vi "LoadObserverControlMatrix_HystSatDrift.vi"(10 "ControlParams-ss-xy":T1={"umax"=3.0, "Ns_obs/cntrl"=0, "du_max"=0.0, "Nbar"=0.0, "Nhyst"=0, "Nsat"=0, "Ndrift+1"=0, "Ki-y"=0.01, "Ns_xff+1"=0, "Ns_yff+1"=0, "Ns_Dx+1"=0, "Ns_Dy+1"=0, "Ki-x"=0.01}) -> (2 "SS FIFO TimeOut?":bool, 3 "ControlParams-ss-xy 2":T1={"umax"=3.0, "Ns_obs/cntrl"=0, "du_max"=0.0, "Nbar"=0.0, "Nhyst"=0, "Nsat"=0, "Ndrift+1"=0, "Ki-y"=0.01, "Ns_xff+1"=0, "Ns_yff+1"=0, "Ns_Dx+1"=0, "Ns_Dy+1"=0, "Ki-x"=0.01})   [LabVIEW 2017]
uses:
  typeDefs/FXPControlParams-ss-xy.ctl
  <vilib>/Platform/TimedLoop/XDataNode/timing_clust.ctl
  <vilib>/Platform/TimedLoop/XDataNode/nitl_modes.ctl
  <vilib>/Platform/TimedLoop/XDataNode/wakeup.ctl
  typeDefs/Bz_bram.ctl
  typeDefs/Lz_bram.ctl
  typeDefs/Kz_bram.ctl
  typeDefs/A_as_vec_bram.ctl
  <vilib>/rvi/interface/RandomDataEmulation/niFpgaRandomDataHandleErrors.vi
  <vilib>/rvi/DataTransferAndStorage/Container/Common/niFpgaContainerExecOnDevCompGetState.vi
  <vilib>/rvi/Emulation/niFpgaEmulationIsFPGAContextNoSignature.vi
  <vilib>/rvi/DataTransferAndStorage/Container/Common/niFpgaContainerGetUniqueNameForEmu.vi
  <vilib>/rvi/Emulation/niFpgaProcessEmulError.vi
  <vilib>/rvi/Emulation/niFpgaSctlEmulationGetInTimedLoop.vi
  <vilib>/rvi/errors/nirviReportUnexpectedCaseInternalError (U32).vi
  <vilib>/rvi/Memory/Memory_Emulation/niFpgaMemoryEmulationCacheClearOnFirstRun.vi
  <vilib>/rvi/Memory/Memory_Emulation/nirvimemoryEmulationManagerCache_MakeExclusive.vi
  <vilib>/rvi/Memory/Memory_Emulation/niFpgaMemoryEmulationValidateCache.vi
  <vilib>/rvi/Memory/Memory_Emulation/nirvimemoryEmulationManagerCache_InsertValue.vi
  <vilib>/Utility/error.llb/Clear Errors.vi
  <vilib>/rvi/Memory/Memory_Emulation/nirvimemoryEmulationManagerCache_ReleaseExclusive.vi
  <vilib>/rvi/Memory/Memory_Emulation/nirvimemoryEmulationManagerCache_GetValue.vi
  <vilib>/rvi/Memory/Memory_Emulation/nirvimemoryEmulationManagerCache_SetValue.vi
  <vilib>/rvi/Emulation/niFpgaSctlEmulationResourceMgr.vi
  <vilib>/rvi/Emulation/niFpgaEmulationReportErrorSimple.vi
  <vilib>/rvi/Emulation/niFpgaGetClockAttributes.vi
  <vilib>/rvi/Emulation/niFpgaCriticalErrorInLSC.vi
  <vilib>/rvi/Memory/Memory_Emulation/nirvimemoryFastEmulation.vi
  <vilib>/rvi/Memory/Memory_Emulation/nirvimemoryEmulation.vi
  <vilib>/rvi/DataTransferAndStorage/Container/XNode/niFpgaContainer.xnode
  <vilib>/rvi/interface/RandomDataEmulation/nirviRandomDataFpgaReadWriteTemplate.vi
  <vilib>/rvi/Memory/Memory_Emulation/niFpgaMemoryEmulationRefIn.vi
  <vilib>/Platform/TimedLoop/XDataNode/XDataNode.xnode
  <vilib>/Platform/TimedLoop/XDataNode/XDNodeRunTimeDep.lvlib
panel:
  # "NOTE: Ns is the number of states in the plant. The number of states in the \nobserver is Ns+1. Thus, for B, L, C, and A, we use NS+1. For K and Xss, we use Ns\nbecause the controller does not operate on the disturbance state, Xd."
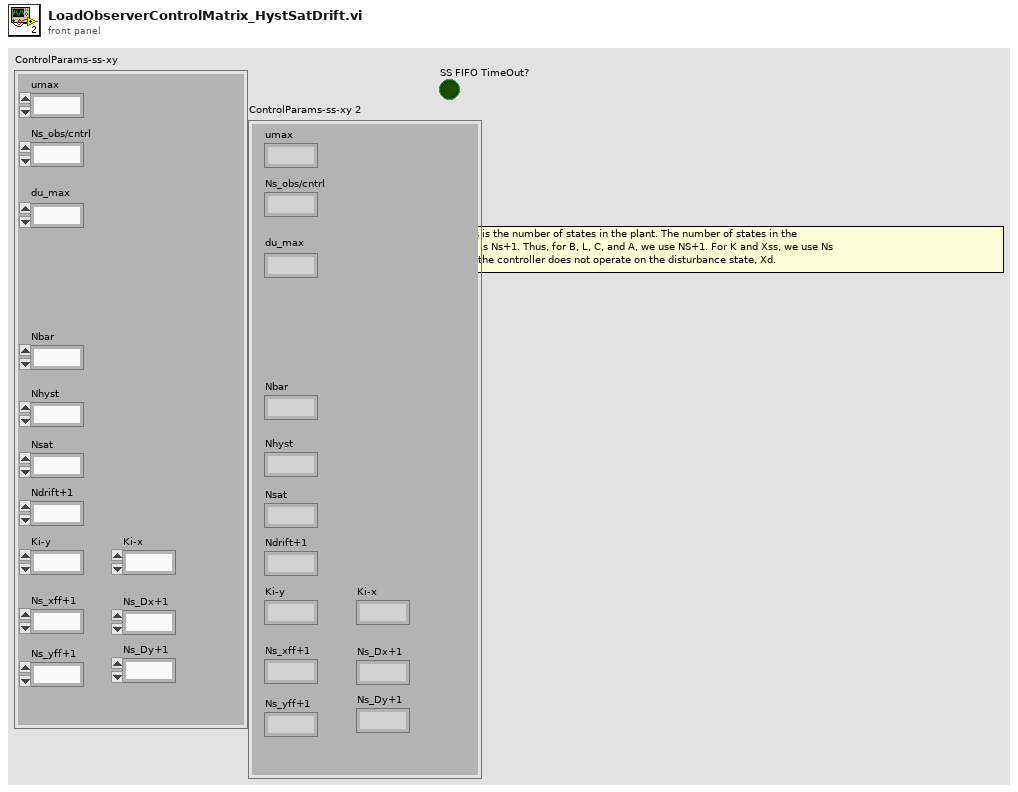
[diagram p1: front panel]
types:
  T1 = typedef "FXPControlParams-ss-xy.ctl" = cluster{"umax":fxp<+/-,18,5>, "Ns_obs/cntrl":u8, "du_max":fxp<+/-,18,5>, "Nbar":fxp<+/-,32,5>, "Nhyst":u8, "Nsat":u8, "Ndrift+1":u8, "Ki-y":sgl, "Ns_xff+1":u8, "Ns_yff+1":u8, "Ns_Dx+1":u8, "Ns_Dy+1":u8, "Ki-x":sgl}
  T2 = typedef "Bz_bram.ctl" = refnum<k21>
  T3 = typedef "Lz_bram.ctl" = refnum<k21>
  T4 = typedef "Kz_bram.ctl" = refnum<k21>
  T5 = typedef "A_as_vec_bram.ctl" = refnum<k21>
  T6 = typedef "XDNodeRunTimeDep.lvlib/timing_clust.ctl" = cluster{"Expected End [f-1]":u64, "Actual End [f-1]":u64, "Finished Late? [f-1]":bool, "Expected End [i-1]":u64, "Actual End [i-1]":u64, "Finished Late? [i-1]":bool, "Expected Start [i]":u64, "Actual Start [i]":u64, "Expected Start [f]":u64, "Actual Start [f]":u64, "Source Name":string, "Structure Name":string, "Period":i64, "Deadline":i64, "Offset":i64, "Start":i64, "Priority":i32, "Timeout":i32, "Mode":T7, "Wakeup Reason":T8, "Error":errorcluster, "Source Type":string, "Secondary Source Type":string, "Global End Time":u64, "Global Start Time":u64, "Frame Duration":u64, "Iteration Duration":u64, "Assigned CPU":i32, "I/O Scan Engine Mode":u32}
  T7 = typedef "XDNodeRunTimeDep.lvlib/nitl_modes.ctl" = enum32{"No Change", "Process missed periods, maintain original phase", "Discard missed periods, maintain original phase", "Process missed periods, ignore original phase", "Discard missed periods, ignore original phase"}
  T8 = typedef "XDNodeRunTimeDep.lvlib/wakeup.ctl" = enum32{"Normal", "Aborted", "Asynchronous wakeup", "Timing source error", "Timed loop error", "Timeout"}
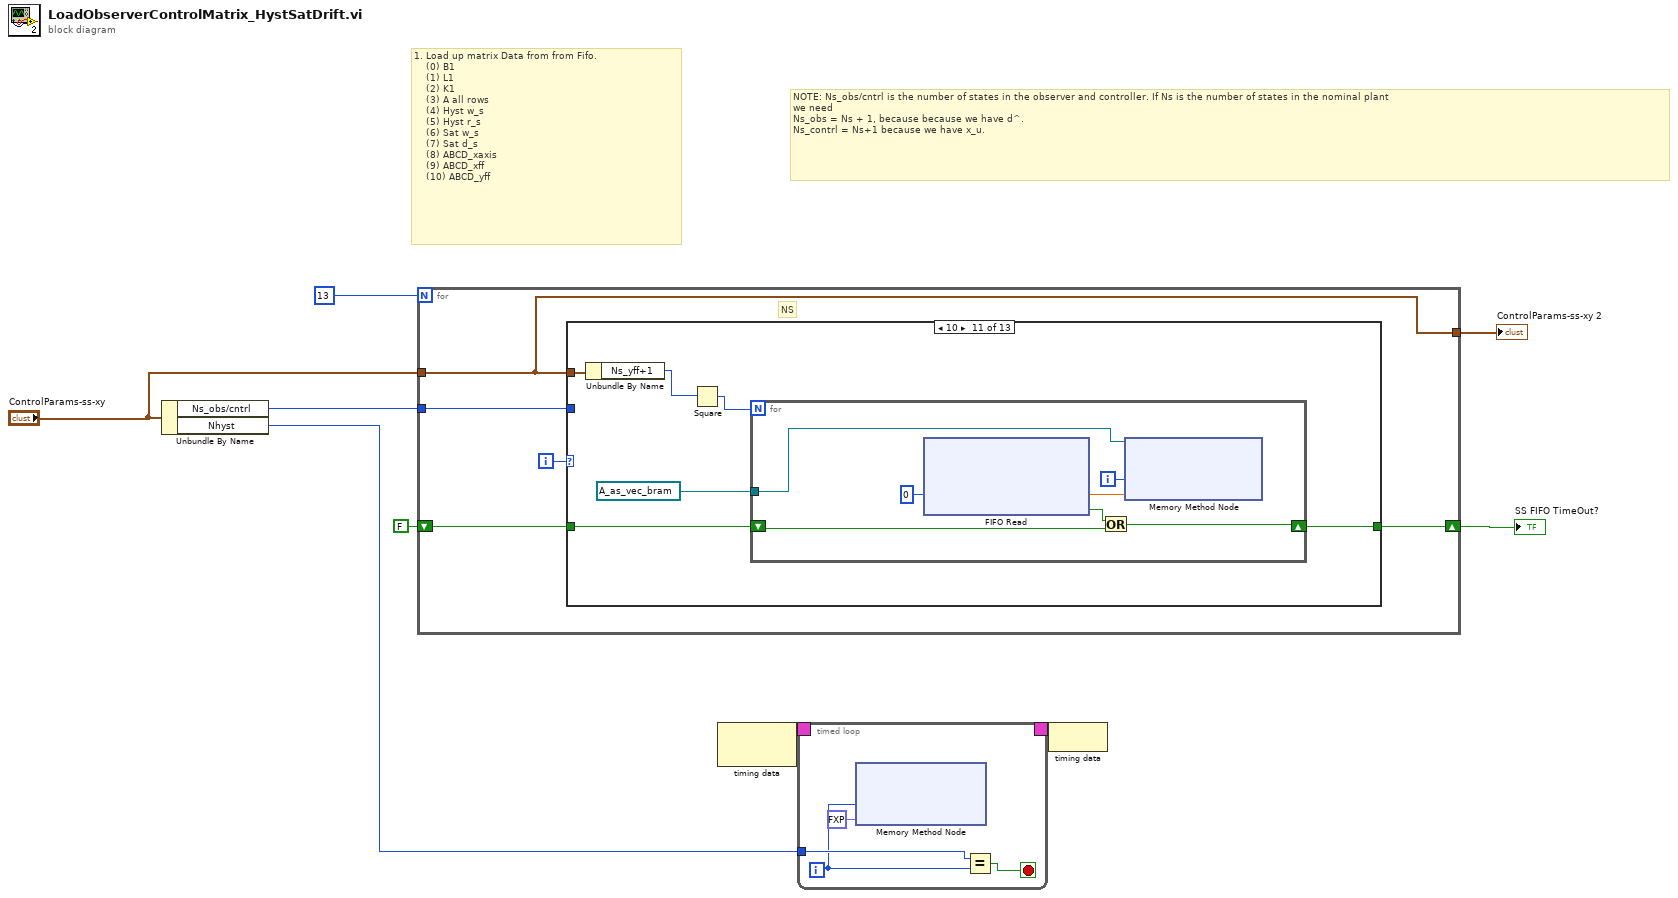
[diagram p0: block diagram]
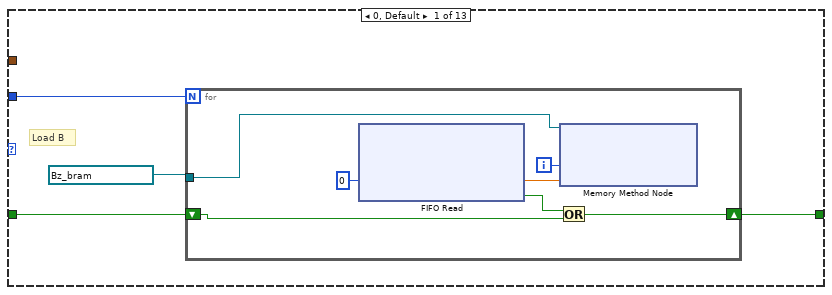
[diagram p2: hidden frame]
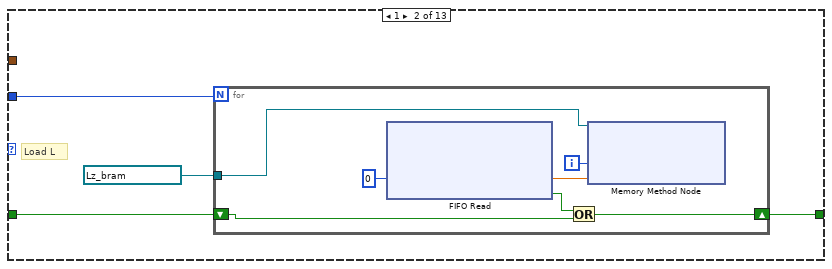
[diagram p3: hidden frame]
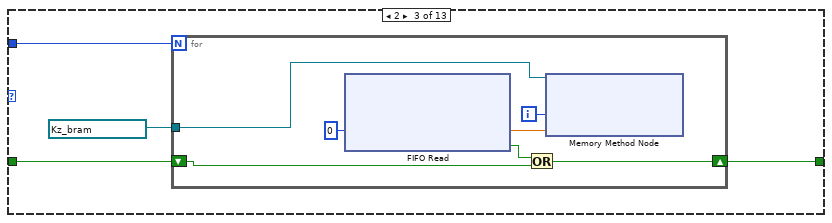
[diagram p4: hidden frame]
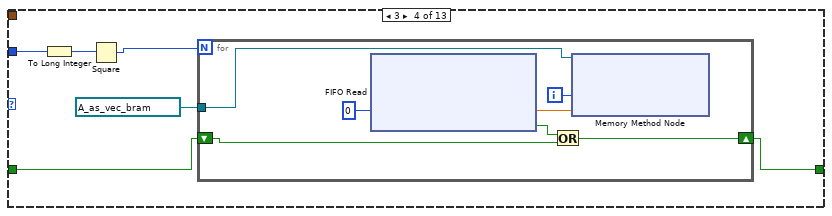
[diagram p5: hidden frame]
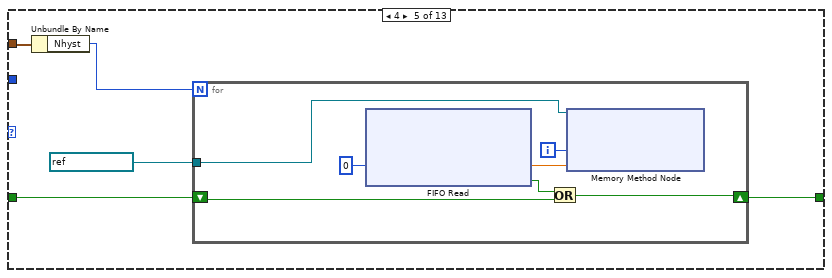
[diagram p6: hidden frame]
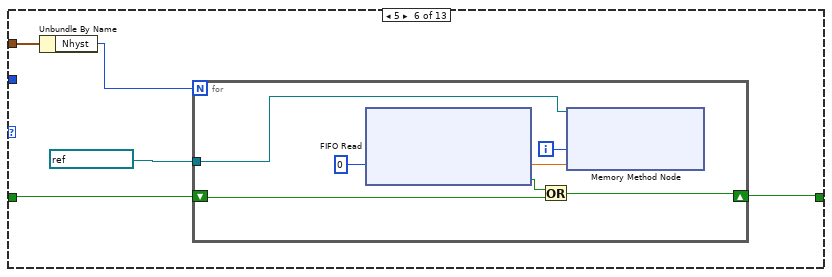
[diagram p7: hidden frame]
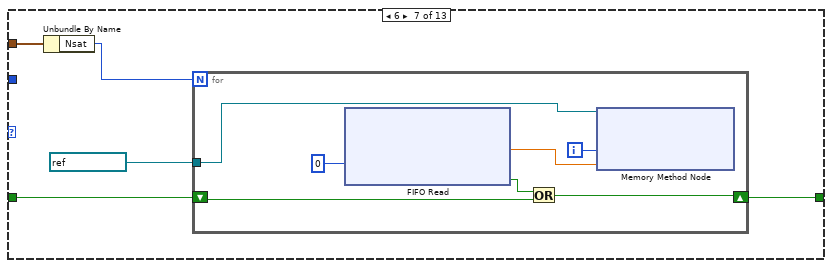
[diagram p8: hidden frame]
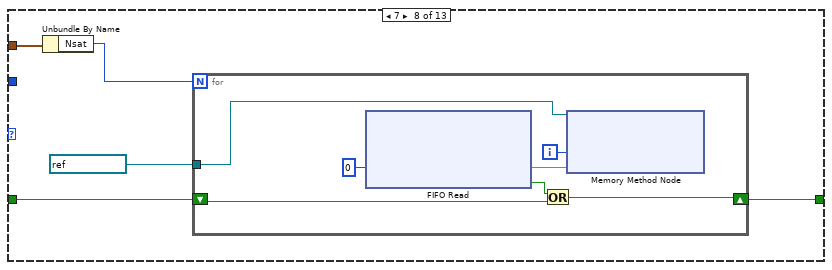
[diagram p9: hidden frame]
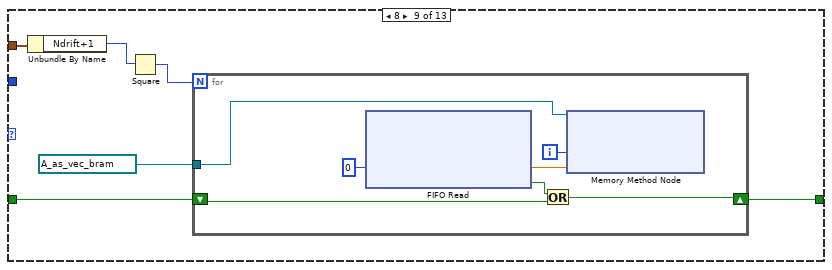
[diagram p10: hidden frame]
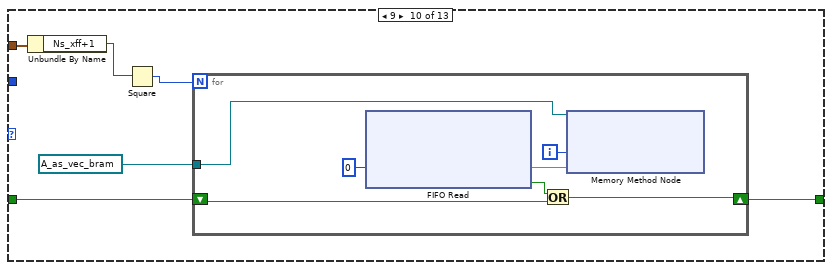
[diagram p11: hidden frame]
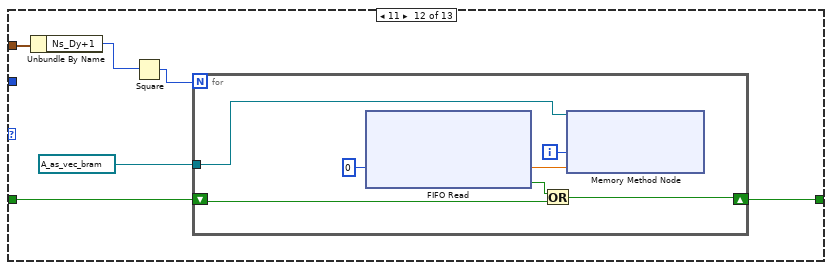
[diagram p12: hidden frame]
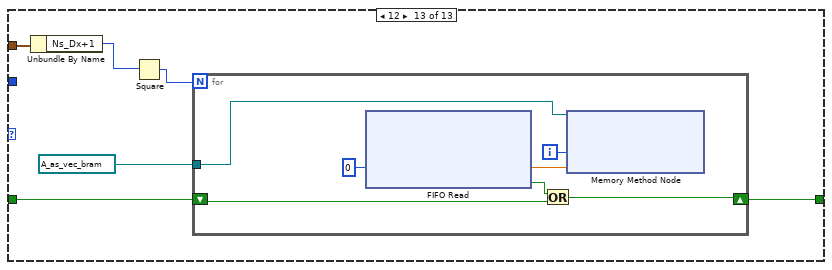
[diagram p13: hidden frame]
diagram:
  # "NOTE: Ns_obs/cntrl is the number of states in the observer and controller. If Ns is the number of states in the nominal plant\nwe need\nNs_obs = Ns + 1, because because we have d^. \nNs_contrl = Ns+1 because we have x_u."
  # "1. Load up matrix Data from from Fifo.\n    (0) B1\n    (1) L1\n    (2) K1 \n    (3) A all rows\n    (4) Hyst w_s\n    (5) Hyst r_s\n    (6) Sat w_s\n    (7) Sat d_s\n    (8) ABCD_xaxis\n    (9) ABCD_xff\n    (10) ABCD_yff"
  n1 = Unbundle By Name("ControlParams-ss-xy") -> ("Ns_obs/cntrl"=w4:u8, "Nhyst"=w3:u8)
  n2 = for {
    N: i16 13 -> [_]
    tunnel: w4 -> [w13]
    shift-right: [w11] -> w7
    shift-left: FALSE -> [w12]
    tunnel: "ControlParams-ss-xy" -> [w10]
    tunnel: [w10] -> w1
    i -> [w14]
    # "NS"
    n3 = case shown="10" w14 {
      tunnel: w13 -> [w18 w26 w40 w49 _ _ _ _ _ _ _ _ _]
      tunnel: w12 -> [w16 w28 w37 w50 w64 w76 w88 w100 w113 w126 w139 w152 w165]
      tunnel: [w15 w27 w38 w51 w65 w77 w89 w101 w114 w127 w140 w153 w166] -> w11
      tunnel: w10 -> [_ _ _ _ w62 w74 w86 w98 w111 w124 w137 w150 w163]
      frame 0, Default {
        # "Load B"
        n4 = for {
          N: w18 -> [_]
          tunnel: T2 "Bz_FXP_col1" ("Memory") -> [w23]
          shift-right: [w20] -> w15
          shift-left: w16 -> [w19]
          i -> [w22]
          n5 = xnode ("FIFO Read")("Timeout"=i16 0) -> ("Element"=w25:sgl, "Timed Out?"=w21:bool)  [unwired: 1 in, 1 out]
          n6 = Or(x=w21, y=w19) -> (x .or. y?=w20:bool)
          n7 = xnode ("Memory Method Node")("Address"=w22, "Data"=w25, "Memory In"=w23) -> ()  [unwired: 1 out]
        }
      }
      frame 1 {
        # "Load L"
        n8 = for {
          N: w26 -> [_]
          tunnel: T3 "L_FXP_col1" ("Memory") -> [w34]
          shift-right: [w31] -> w27
          shift-left: w28 -> [w30]
          i -> [w33]
          n9 = xnode ("FIFO Read")("Timeout"=i16 0) -> ("Element"=w36:sgl, "Timed Out?"=w32:bool)  [unwired: 1 in, 1 out]
          n10 = Or(x=w32, y=w30) -> (x .or. y?=w31:bool)
          n11 = xnode ("Memory Method Node")("Address"=w33, "Data"=w36, "Memory In"=w34) -> ()  [unwired: 1 out]
        }
      }
      frame 2 {
        n12 = for {
          N: w40 -> [_]
          tunnel: T4 "K_FXP_row1" ("Memory") -> [w45]
          shift-right: [w42] -> w38
          shift-left: w37 -> [w41]
          i -> [w44]
          n13 = xnode ("FIFO Read")("Timeout"=i16 0) -> ("Element"=w47:sgl, "Timed Out?"=w43:bool)  [unwired: 1 in, 1 out]
          n14 = Or(x=w43, y=w41) -> (x .or. y?=w42:bool)
          n15 = xnode ("Memory Method Node")("Address"=w44, "Data"=w47, "Memory In"=w45) -> ()  [unwired: 1 out]
        }
      }
      frame 3 {
        n16 = To Long Integer(number=w49) -> (32bit integer=w48:i32)
        n17 = Square(x=w48) -> (x^2=w53:i32)
        n18 = for {
          N: w53 -> [_]
          tunnel: T5 "AasCol _FXP" ("Memory In") -> [w58]
          shift-right: [w55] -> w51
          shift-left: w50 -> [w54]
          i -> [w57]
          n19 = xnode ("FIFO Read")("Timeout"=i16 0) -> ("Element"=w60:sgl, "Timed Out?"=w56:bool)  [unwired: 1 in, 1 out]
          n20 = Or(x=w56, y=w54) -> (x .or. y?=w55:bool)
          n21 = xnode ("Memory Method Node")("Address"=w57, "Data"=w60, "Memory In"=w58) -> ()  [unwired: 1 out]
        }
      }
      frame 4 {
        n22 = Unbundle By Name(w62) -> ("Nhyst"=w61:u8)
        n23 = for {
          N: w61 -> [_]
          tunnel: refnum<k21> "hyst_w_s" ("Memory In") -> [w70]
          shift-right: [w67] -> w65
          shift-left: w64 -> [w66]
          i -> [w69]
          n24 = xnode ("FIFO Read")("Timeout"=i16 0) -> ("Element"=w72:sgl, "Timed Out?"=w68:bool)  [unwired: 1 in, 1 out]
          n25 = Or(x=w68, y=w66) -> (x .or. y?=w67:bool)
          n26 = xnode ("Memory Method Node")("Address"=w69, "Data"=w72, "Memory In"=w70) -> ()  [unwired: 1 out]
        }
      }
      frame 5 {
        n27 = Unbundle By Name(w74) -> ("Nhyst"=w73:u8)
        n28 = for {
          N: w73 -> [_]
          tunnel: refnum<k21> "hyst_r_s" ("Memory In") -> [w82]
          shift-right: [w79] -> w77
          shift-left: w76 -> [w78]
          i -> [w81]
          n29 = xnode ("FIFO Read")("Timeout"=i16 0) -> ("Element"=w84:sgl, "Timed Out?"=w80:bool)  [unwired: 1 in, 1 out]
          n30 = Or(x=w80, y=w78) -> (x .or. y?=w79:bool)
          n31 = xnode ("Memory Method Node")("Address"=w81, "Data"=w84, "Memory In"=w82) -> ()  [unwired: 1 out]
        }
      }
      frame 6 {
        n32 = Unbundle By Name(w86) -> ("Nsat"=w85:u8)
        n33 = for {
          N: w85 -> [_]
          tunnel: refnum<k21> "sat_w_s" ("Memory In") -> [w94]
          shift-right: [w91] -> w89
          shift-left: w88 -> [w90]
          i -> [w93]
          n34 = xnode ("FIFO Read")("Timeout"=i16 0) -> ("Element"=w96:sgl, "Timed Out?"=w92:bool)  [unwired: 1 in, 1 out]
          n35 = Or(x=w92, y=w90) -> (x .or. y?=w91:bool)
          n36 = xnode ("Memory Method Node")("Address"=w93, "Data"=w96, "Memory In"=w94) -> ()  [unwired: 1 out]
        }
      }
      frame 7 {
        n37 = Unbundle By Name(w98) -> ("Nsat"=w97:u8)
        n38 = for {
          N: w97 -> [_]
          tunnel: refnum<k21> "sat_d_s" ("Memory In") -> [w106]
          shift-right: [w103] -> w101
          shift-left: w100 -> [w102]
          i -> [w105]
          n39 = xnode ("FIFO Read")("Timeout"=i16 0) -> ("Element"=w108:sgl, "Timed Out?"=w104:bool)  [unwired: 1 in, 1 out]
          n40 = Or(x=w104, y=w102) -> (x .or. y?=w103:bool)
          n41 = xnode ("Memory Method Node")("Address"=w105, "Data"=w108, "Memory In"=w106) -> ()  [unwired: 1 out]
        }
      }
      frame 8 {
        n42 = Unbundle By Name(w111) -> ("Ndrift+1"=w109:u8)
        n43 = Square(x=w109) -> (x^2=w110:u8)
        n44 = for {
          N: w110 -> [_]
          tunnel: T5 "ABCD_xaxis" ("Memory In") -> [w119]
          shift-right: [w116] -> w114
          shift-left: w113 -> [w115]
          i -> [w118]
          n45 = xnode ("FIFO Read")("Timeout"=i16 0) -> ("Element"=w121:sgl, "Timed Out?"=w117:bool)  [unwired: 1 in, 1 out]
          n46 = Or(x=w117, y=w115) -> (x .or. y?=w116:bool)
          n47 = xnode ("Memory Method Node")("Address"=w118, "Data"=w121, "Memory In"=w119) -> ()  [unwired: 1 out]
        }
      }
      frame 9 {
        n48 = Unbundle By Name(w124) -> ("Ns_xff+1"=w123:u8)
        n49 = Square(x=w123) -> (x^2=w122:u8)
        n50 = for {
          N: w122 -> [_]
          tunnel: T5 "ABCD_xff" ("Memory In") -> [w132]
          shift-right: [w129] -> w127
          shift-left: w126 -> [w128]
          i -> [w131]
          n51 = xnode ("FIFO Read")("Timeout"=i16 0) -> ("Element"=w134:sgl, "Timed Out?"=w130:bool)  [unwired: 1 in, 1 out]
          n52 = Or(x=w130, y=w128) -> (x .or. y?=w129:bool)
          n53 = xnode ("Memory Method Node")("Address"=w131, "Data"=w134, "Memory In"=w132) -> ()  [unwired: 1 out]
        }
      }
      frame 10 {
        n54 = Unbundle By Name(w137) -> ("Ns_yff+1"=w136:u8)
        n55 = Square(x=w136) -> (x^2=w135:u8)
        n56 = for {
          N: w135 -> [_]
          tunnel: T5 "ABCD_yff" ("Memory In") -> [w145]
          shift-right: [w142] -> w140
          shift-left: w139 -> [w141]
          i -> [w144]
          n57 = xnode ("FIFO Read")("Timeout"=i16 0) -> ("Element"=w147:sgl, "Timed Out?"=w143:bool)  [unwired: 1 in, 1 out]
          n58 = Or(x=w143, y=w141) -> (x .or. y?=w142:bool)
          n59 = xnode ("Memory Method Node")("Address"=w144, "Data"=w147, "Memory In"=w145) -> ()  [unwired: 1 out]
        }
      }
      frame 11 {
        n60 = Unbundle By Name(w150) -> ("Ns_Dy+1"=w149:u8)
        n61 = Square(x=w149) -> (x^2=w148:u8)
        n62 = for {
          N: w148 -> [_]
          tunnel: T5 "ABCD_Dy" ("Memory In") -> [w158]
          shift-right: [w155] -> w153
          shift-left: w152 -> [w154]
          i -> [w157]
          n63 = xnode ("FIFO Read")("Timeout"=i16 0) -> ("Element"=w160:sgl, "Timed Out?"=w156:bool)  [unwired: 1 in, 1 out]
          n64 = Or(x=w156, y=w154) -> (x .or. y?=w155:bool)
          n65 = xnode ("Memory Method Node")("Address"=w157, "Data"=w160, "Memory In"=w158) -> ()  [unwired: 1 out]
        }
      }
      frame 12 {
        n66 = Unbundle By Name(w163) -> ("Ns_Dx+1"=w162:u8)
        n67 = Square(x=w162) -> (x^2=w161:u8)
        n68 = for {
          N: w161 -> [_]
          tunnel: T5 "ABCD_Dx" ("Memory In") -> [w171]
          shift-right: [w168] -> w166
          shift-left: w165 -> [w167]
          i -> [w170]
          n69 = xnode ("FIFO Read")("Timeout"=i16 0) -> ("Element"=w173:sgl, "Timed Out?"=w169:bool)  [unwired: 1 in, 1 out]
          n70 = Or(x=w169, y=w167) -> (x .or. y?=w168:bool)
          n71 = xnode ("Memory Method Node")("Address"=w170, "Data"=w173, "Memory In"=w171) -> ()  [unwired: 1 out]
        }
      }
    }
  }
  "SS FIFO TimeOut?" <- w7
  "ControlParams-ss-xy 2" <- w1
  n72 = node-c288() -> (w6:T6)  [unwired: 1 in]
  n73 = timed-loop {
    timing: w6 -> [_]
    timing-out: [_] -> w5
    tunnel: w3 -> [w176]
    i -> [w174]
    stop <- w177 stop-if-true
    n74 = xnode ("Memory Method Node")("Address"=w174, "Data"=fxp<+/-,16,5> 0.0) -> ()  [unwired: 1 in, 1 out]
    n75 = Equal?(x=w176, y=w174) -> (x = y?=w177:bool)
  }
  n76 = node-c288(w5) -> ()
